vi "Sensor Data (Single Reading).vi"(8 "error in (no error)":errorcluster, 9 "Data Source (0:Kelvin)":u16(ring) items=["Kelvin", "Celsius", "Sensor Units"], 10 "Sensor Input (0:A)":u16(ring) items=["A", "B"], 11 "VISA resource name":refnum<visa-resource-name>) -> (0 "error out":errorcluster, 2 "Sensor Data":dbl format="%.4f", 3 "VISA resource name out":refnum<visa-resource-name>)   [LabVIEW 2019, in "Lake Shore 325.lvlib"]
doc: "Reads and returns a single sensor reading from the instrument."
uses:
  Lake Shore 325.lvlib
  Instance           1 36Saved   Sensor Data (Single Reading) .vi
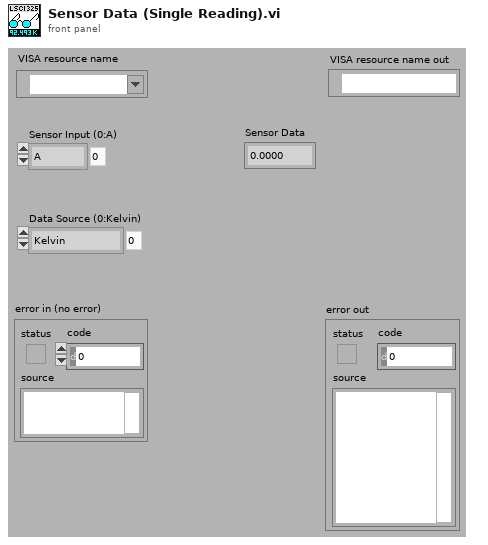
[diagram p1: front panel]
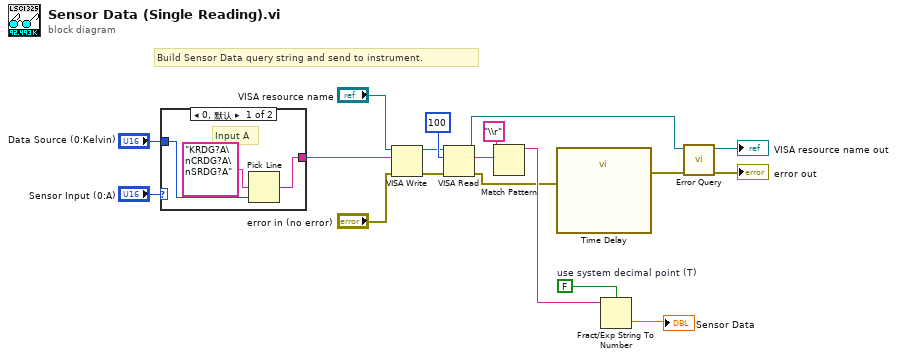
[diagram p0: block diagram]
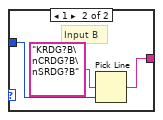
[diagram p2: hidden frame]
diagram:
  w8 = FALSE  # use system decimal point (T)
  # "Build Sensor Data query string and send to instrument."
  n1 = case shown="0, 默认" "Sensor Input (0:A)" {
    tunnel: "Data Source (0:Kelvin)" -> [w20 w22]
    tunnel: [w19 w23] -> w3
    frame 0, Default {
      # "Input A"
      n2 = Pick Line(multi-line string="KRDG?A\nCRDG?A\nSRDG?A", line index=w20) -> (output string=w19:string)  [unwired: 1 in]
    }
    frame 1 {
      # "Input B"
      n3 = Pick Line(multi-line string="KRDG?B\nCRDG?B\nSRDG?B", line index=w22) -> (output string=w23:string)  [unwired: 1 in]
    }
  }
  n4 = VISA Write(VISA resource name="VISA resource name", write buffer=w3, error in (no error)="error in (no error)") -> (VISA resource name out=w10:refnum<visa-resource-name>, error out=w9:errorcluster)  [unwired: 1 out]
  n5 = VISA Read(VISA resource name=w10, byte count=100, error in (no error)=w9) -> (VISA resource name out=w14:refnum<visa-resource-name>, read buffer=w12:string, error out=w1:errorcluster)  [unwired: 1 out]
  n6 = Match Pattern(string=w12, regular expression="\\r") -> (before substring=w6:string)  [unwired: 1 in, 3 out]
  n7 = call "Time Delay"("error in (no error)"=w1) -> ("error out"=w2:errorcluster)  [unwired: 10 in]
  n8 = Fract/Exp String To Number(use system decimal point (T)=w8, string=w6) -> (number=→"Sensor Data":dbl)  [unwired: 2 in, 1 out]
  n9 = call "Error Query.vi"("error in (no error)"=w2, "VISA resource name"=w14) -> ("error out"=→"error out":errorcluster, "VISA resource name out"=→"VISA resource name out":refnum<visa-resource-name>)  [unwired: 7 in, 1 out]
